vi "SetupInterfArrDev.vi"(8 "error in (no error)":errorcluster caption="entrée d'erreur (pas d'erreur)", 9 "Experiment.lvclass":refnum<class "Experiment.lvclass">=refnum, 10 "DevID":i32, 11 "Interface en entrée":refnum<class "Interface.lvclass"> caption="Interface Class in") -> (0 "error out":errorcluster caption="sortie d'erreur", 2 "CurveParamsOut":T1[](array[typedef]), 3 "Interface en sortie":refnum<class "Interface.lvclass"> caption="DNL_LabVIEW Object out")   [LabVIEW 2019, in "Interface.lvclass"]
uses:
  Interface.lvclass
  Experiment Class/Experiment.lvclass
  DevicesClass/Tools/Tools.lvclass
  CurveSetup.ctl
  SetupInterfStates.ctl
  Interface.lvclass/Interface.ctl
  2DGraphSetup.ctl
panel:
  in  "Apply All":bool
  out "InstrPref":string
  in  "SaveCurveParDef":bool
  out "GraphConfig":i32
  out "2D Scan":bool
  in  "2D Plot Act":bool caption="2D Plot"
  out "Fill Line First":bool
  in  "2D Plot":bool
  in  "2D YScanPar":u16(ring) caption="Y Parameter"
  in  "2D XScanPar":u16(ring) caption="X Parameter"
  in  "Data Only":bool
  out "GraphIndex":i32
  in  "YScale":u32(ring) items=["Left 1", "Left 2", "Left 3", "Right 1", "Right 2", "Right 3"]
  in  "X Scale":u32(ring) items=["Bottom", "Top"]
  in  "SaveCurvePar":bool
  in  "DisplayName":string
  in  "Visible":bool
  out "CrvParOut":T1[](array[typedef])
  out "NomDon":string[](array[string])=["RTêta;", "X&Y;"]
  out "VarParams":string[][](array[string])
  in  "AutoColor":bool caption="Use Automatic Color"
  out "Graphe XY":cluster{dbl, dbl}[](graph)
  in  "ScanParam":u16(ring) caption="Scan Parameter" items=["Tools.Ind Point(Point)", "Tools_1.Ind Point(Point)"]
  in  "YScaleName":string
  in  "XScaleName":string
  in  "Graph Window":i32(ring) items=["Graph 0", "No Graph", "New Graph Window For Each Curve", "New Graph Window For Each Scan"]
  in  "stop":bool
  in  "Curve List":i32(listbox)
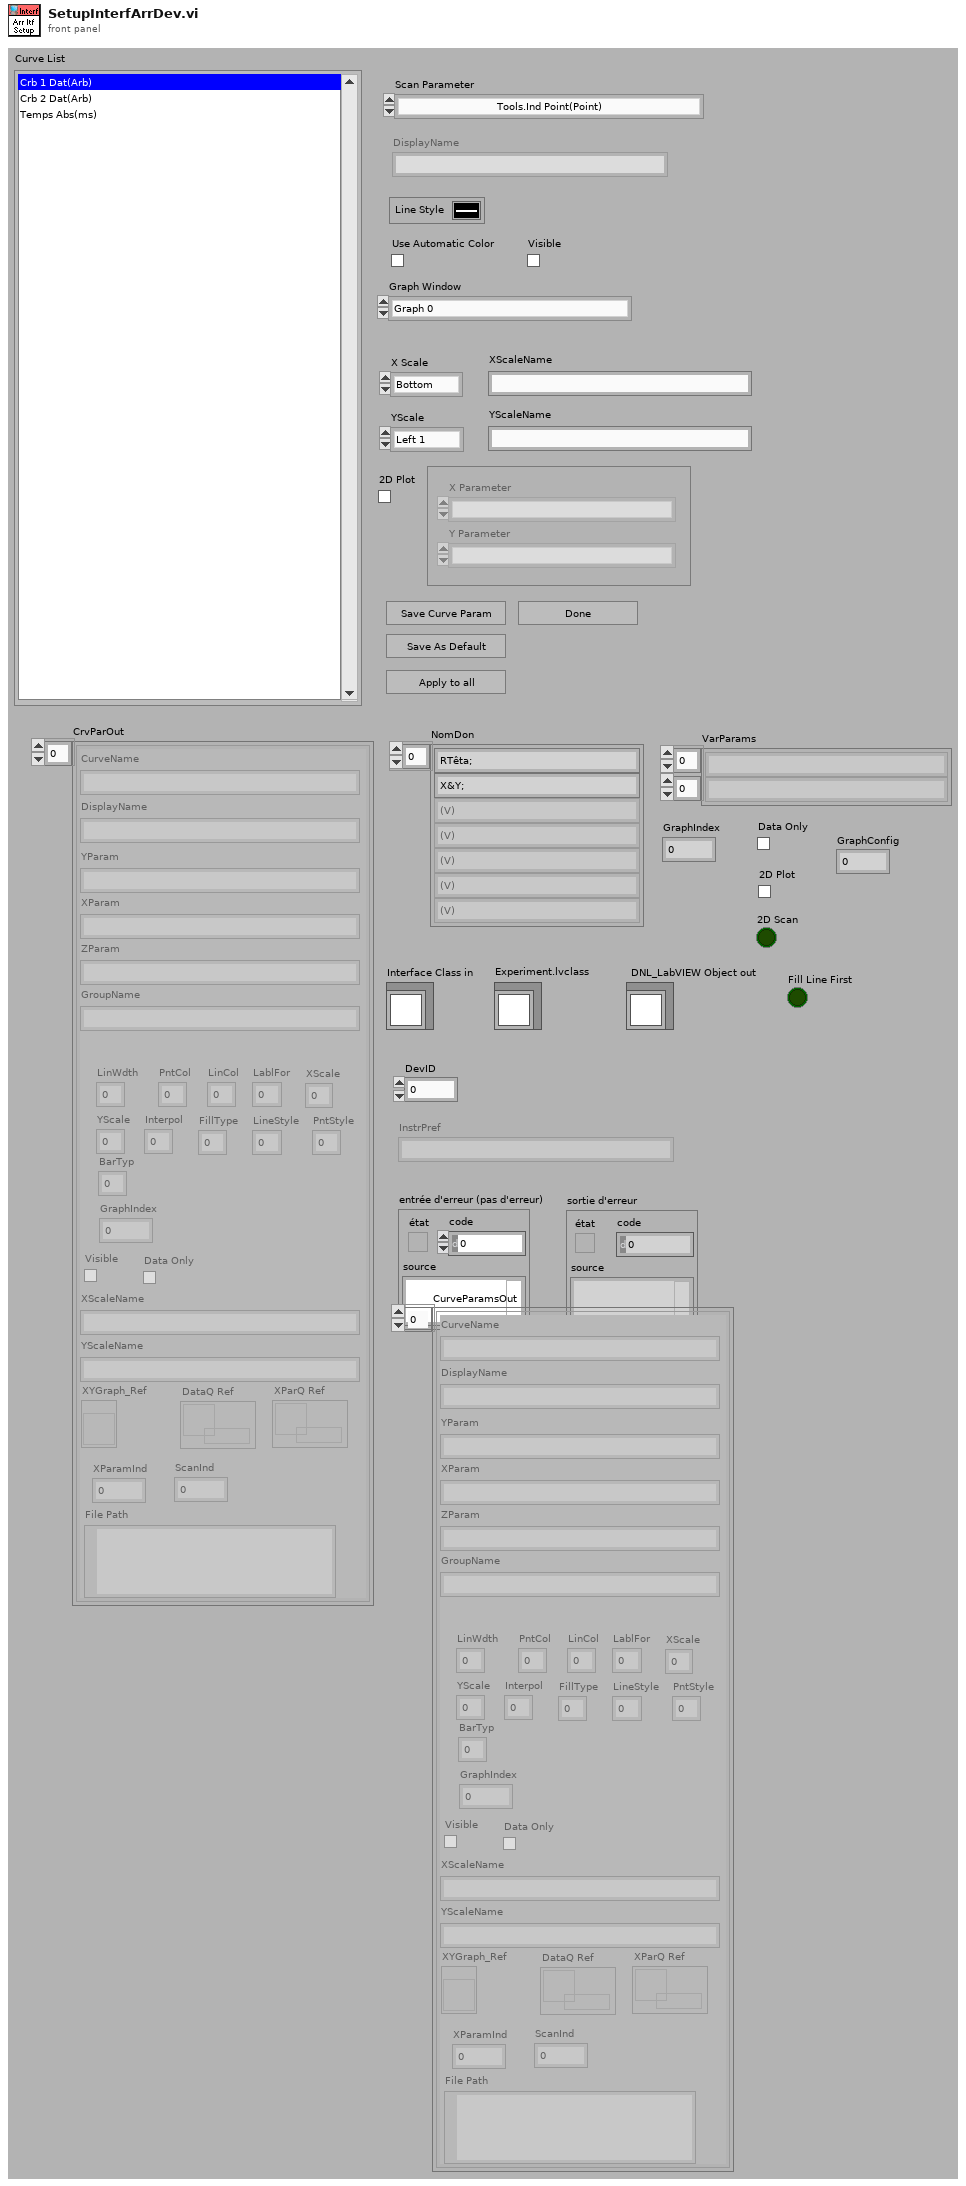
[diagram p1: front panel]
types:
  T1 = typedef "Interface.lvclass/CurveSetup.ctl" = cluster{"CurveName":string, "YParam":string, "XParam":string, "ZParam ":string, "GroupName":string, "LinWdth":u8, "PntCol":u32, "LinCol":u32, "LablFor":u8, "XScale":u32, "YScale":u32, "Interpol":u8, "DisplayName":string, "FillType":i16, "LineStyle":u8, "PntStyle":u8, "BarTyp":u8, "GraphIndex":i32, "Visible":bool, "XScaleName":string, "YScaleName":string, "XYGraph_Ref":refnum<vi>, "Data Only":bool, "DataQ Ref":refnum<queue>, "XParQ Ref":refnum<queue>, "XParamInd":i32, "ScanInd":i32, "File Path":path}
  T2 = typedef "SetupInterfStates.ctl" = enum16{"InitProg", "ReadMeasPar", "ReadCurvePar", "ReadGraphPar", "GetScaleName", "ChgScaleName", "ChngGraphConf", "2D Graph", "SaveParams", "SaveParamsDef", "ApplyAll", "ArrDevSetup", "Stop"}
  T3 = enum16{"Enable", "Disable", "DisAndGrayed", "ReinitToDefVal"}
  T4 = enum16{"Enable", "Disable", "DisAndGrayed", "ReinitToDefVal", "EnumElementsArr"}
  T5 = typedef "2DGraphSetup.ctl" = cluster{"ZDataIndex":i32, "XParIndex":i32, "YParIndex":i32, "FillLineFirst":bool, "2DGraphIndex":i32, "XParQ Ref":refnum<queue>, "YParQ Ref":refnum<queue>, "DataQRefs":refnum<queue>[], "CurveName":string, "XparInstrInd":i32, "YparInstrInd":i32, "Active":bool}
  T6 = enum32{"Invalid", "Standard", "Closed", "Hidden", "Minimized", "Maximized"}
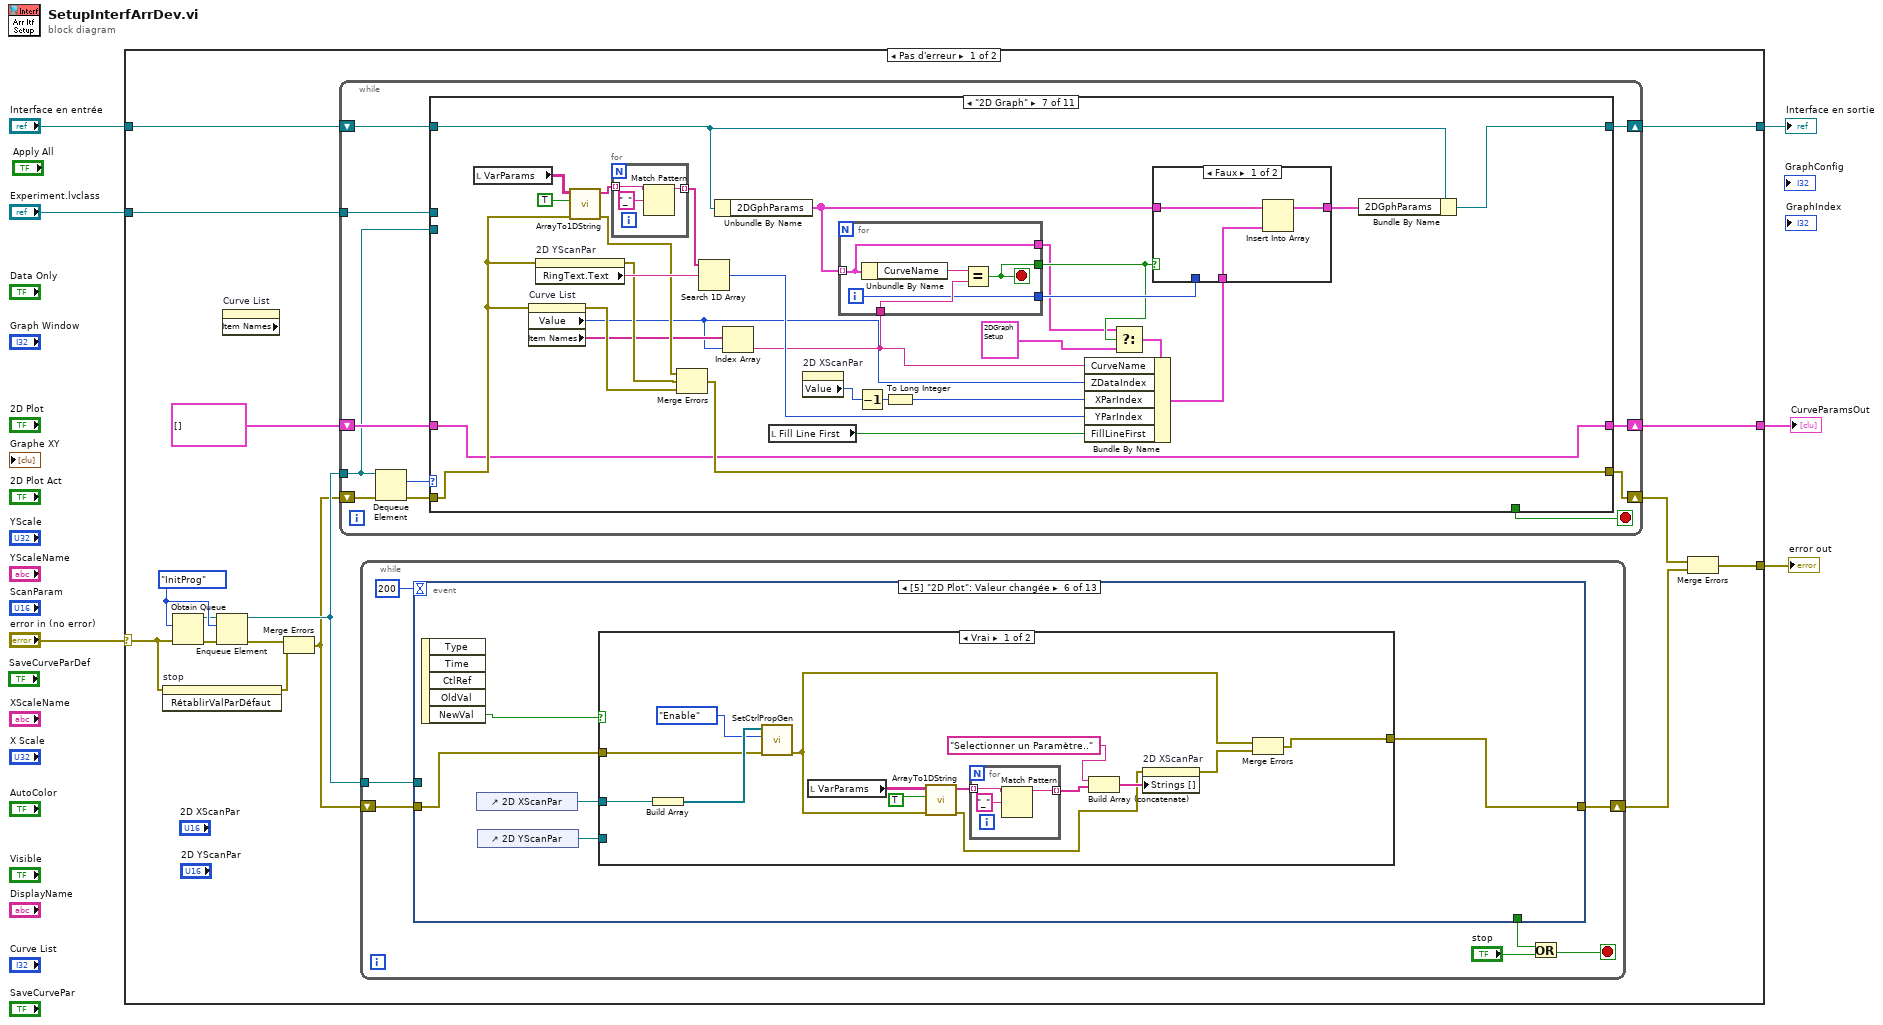
[diagram p0: block diagram]
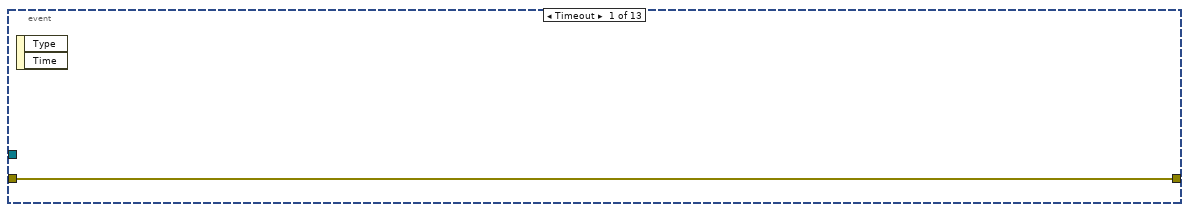
[diagram p2: hidden frame]
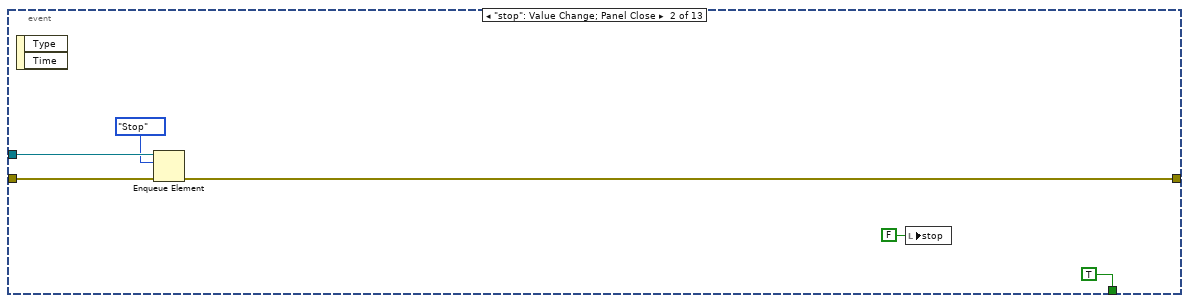
[diagram p3: hidden frame]
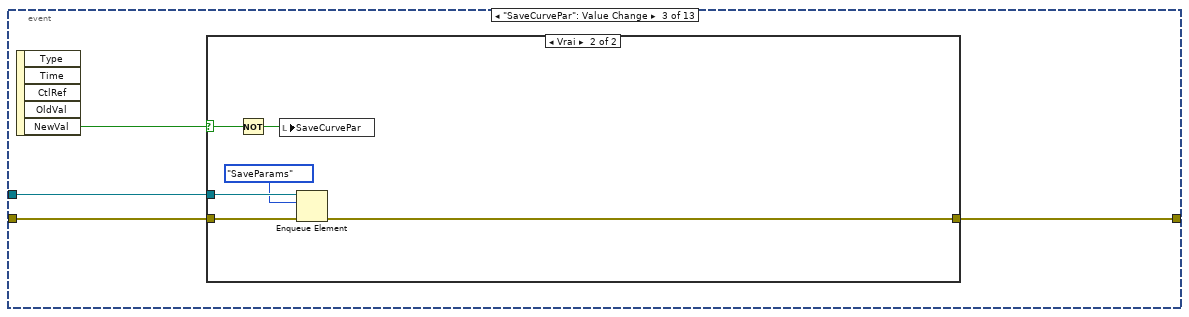
[diagram p4: hidden frame]
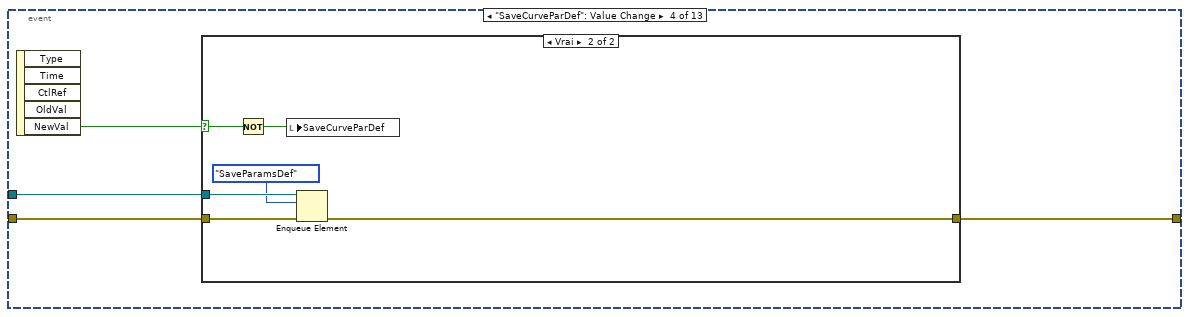
[diagram p6: hidden frame]
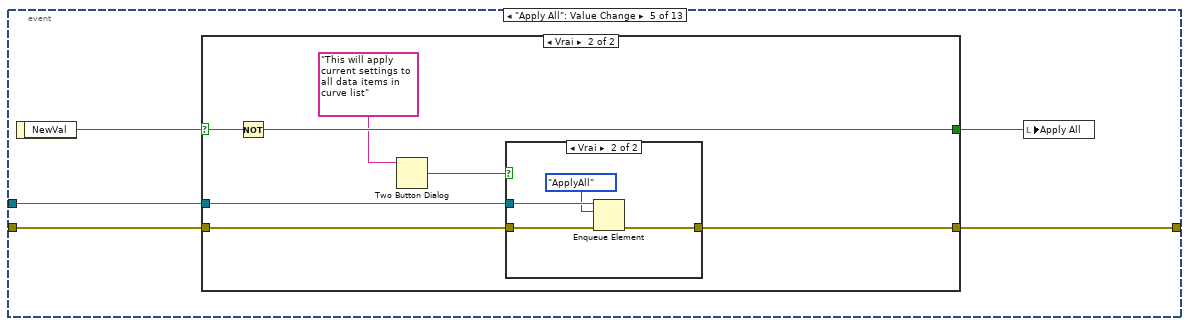
[diagram p8: hidden frame]
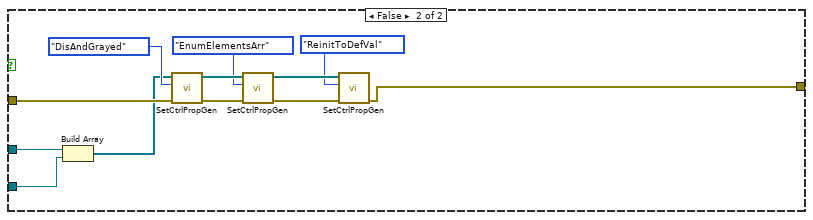
[diagram p11: hidden frame]
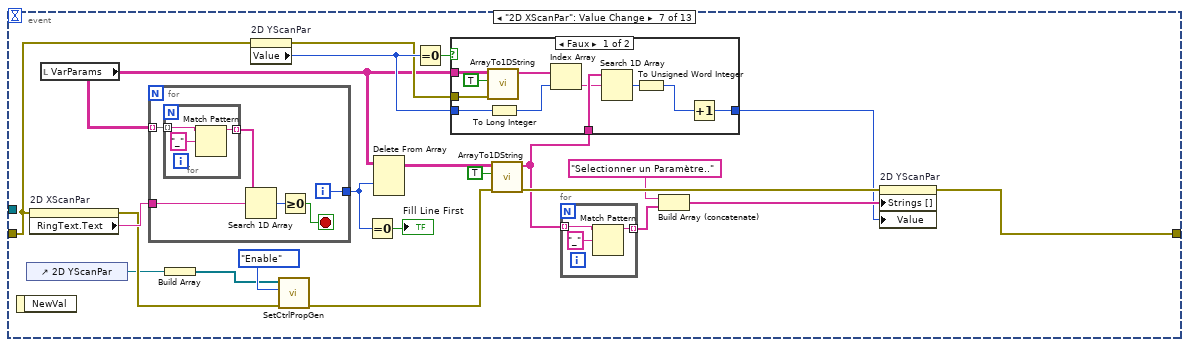
[diagram p12: hidden frame]
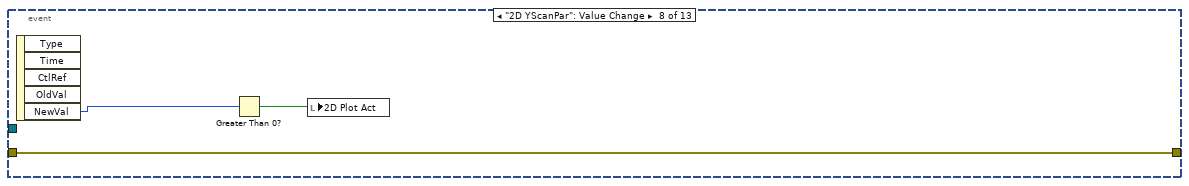
[diagram p14: hidden frame]
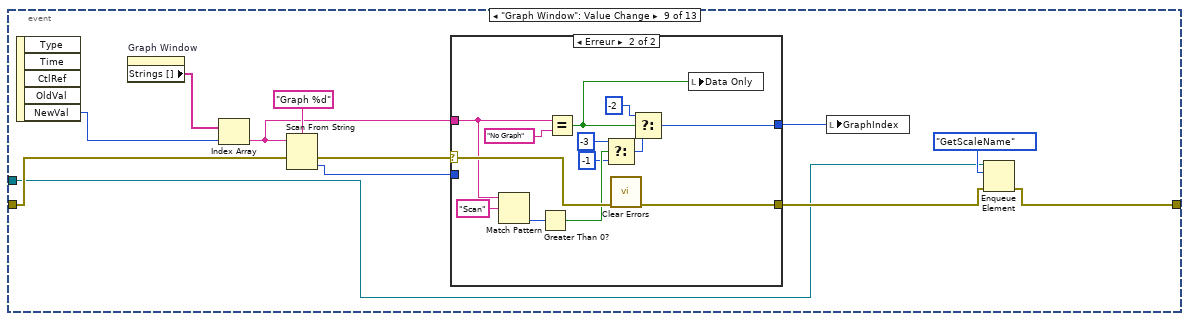
[diagram p15: hidden frame]
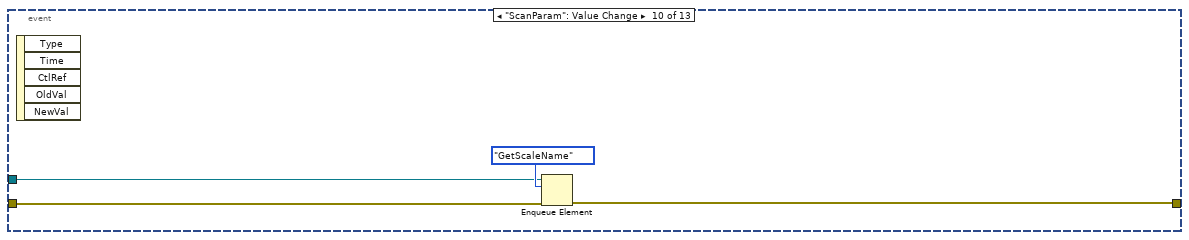
[diagram p17: hidden frame]
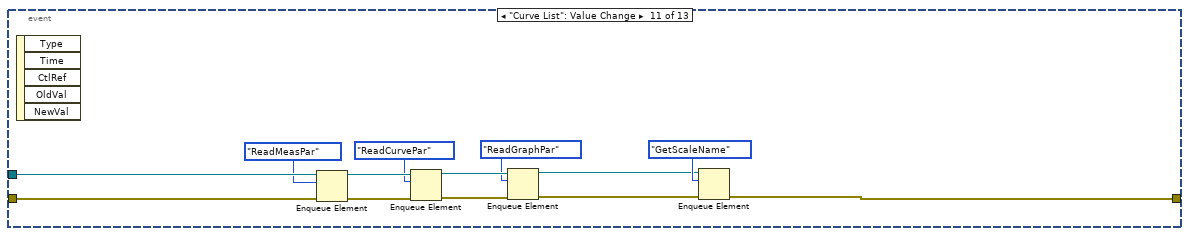
[diagram p18: hidden frame]
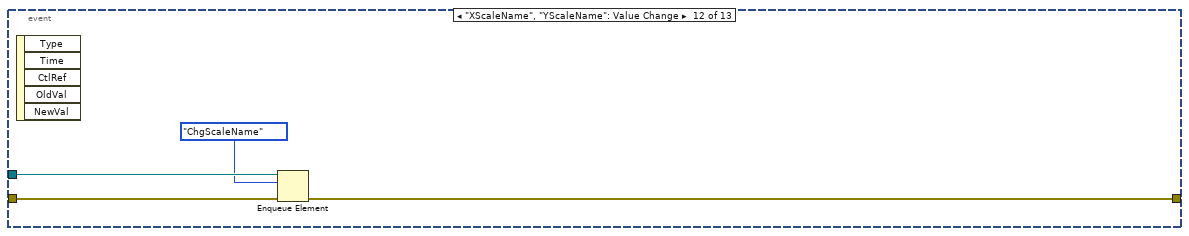
[diagram p19: hidden frame]
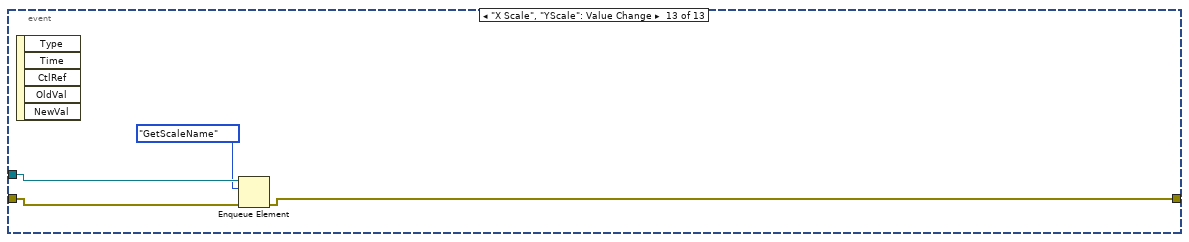
[diagram p20: hidden frame]
diagram:
  n1 = case shown="Pas d'erreur" "error in (no error)" {
    selector: "error in (no error)" -> [w17 w791]
    tunnel: [w10 w791] -> w5
    tunnel: "Interface en entrée" -> [w13 w790]
    tunnel: [w8 w790] -> w3
    tunnel: "Experiment.lvclass" -> [w9 _]
    tunnel: [w7 _] -> w1
    frame No Error {
      w22 = SetupInterfStates."InitProg" ("Énum")
      n2 = invoke on="stop" class="Bool (strict)" method="RétablirValParDéfaut"(error in=w17) -> (error out=w15:errorcluster)  [unwired: 2 in, 2 out]
      n3 = Obtain Queue(element data type=w22, error in (no error)=w17) -> (queue out=w21:refnum<queue>, error out=w20:errorcluster)  [unwired: 3 in, 1 out]
      n4 = Enqueue Element(queue=w21, element=w22, error in (no error)=w20) -> (queue out=w19:refnum<queue>, error out=w16:errorcluster)  [unwired: 1 in, 1 out]
      n5 = property on="Curve List" class="LstDér (strict)" props=["Item Names"]() -> ()  [unwired: 2 in, 3 out]
      n6 = Merge Errors(w16, w15) -> (w14:errorcluster)
      n7 = while {
        shift-right: [w217] -> w11
        shift-left: w14 -> [w222]
        tunnel: w19 -> [w214]
        shift-right: [w218] -> w8
        shift-left: w13 -> [w221]
        shift-right: [w216] -> w7
        shift-left: T1[] [] ("CurveParamsOut") -> [w215]
        tunnel: w9 -> [w213]
        stop <- w219 stop-if-true
        n8 = Dequeue Element(queue=w214, error in (no error)=w222) -> (element=w223:T2, error out=w220:errorcluster)  [unwired: 1 in, 2 out]
        n9 = case shown="\"2D Graph\"" w223 {
          tunnel: w221 -> [w227 w307 w308 w371 w443 w474 w501 w587 w614 w718 w784]
          tunnel: w220 -> [w264 w301 w331 w387 w454 w481 w503 w589 w615 w691 w778]
          tunnel: [FALSE _ _ _ _ _ _ _ _ _ TRUE] -> w219
          tunnel: [w226 w307 w308 w371 w443 w470 w500 w588 w606 w729 w784] -> w218
          tunnel: [w259 w297 w316 w358 w455 w468 w495 w590 w608 w695 w782] -> w217
          tunnel: [w225 w296 w329 w384 w465 w484 w492 w529 w605 w694 w783] -> w216
          tunnel: w215 -> [_ w296 w329 w384 w465 w484 w492 w591 w616 w692 w783]
          tunnel: w214 -> [_ _ _ _ _ _ _ w586 w613 w712 _]
          tunnel: w213 -> [w254 _ _ _ _ _ _ _ _ _ _]
          frame "InitProg", Default {
            w267 = 1 ("indice")
            # "reads the available CurveSetup or get default values"
            n10 = invoke on="2D Plot" class="Bool (strict)" method="RétablirValParDéfaut"(error in=w264) -> (error out=w251:errorcluster)  [unwired: 2 in, 2 out]
            n11 = Unbundle By Name(w227) -> ("GraphConfig"=w255:i32, "CurvesSetup"=w233:T1[], "IndCourbe"=w253:i64)
            n12 = local write "GraphConfig"(w255) -> ()
            n13 = call "ArrayDevScan.vi"("error in"=w251, "IndCourbe"=w253, "DevID"="DevID", "Experiment.lvclass In"=w254) -> ("error out"=w248:errorcluster, "ArrNomDon"=→"NomDon":string[], "ArrVarParsOut"=w249:string[][], "ArrScan list"=w245:string[], "ArrVarPar list"=w246:string[])  [unwired: 2 in, 1 out]
            "VarParams" <- w249
            n14 = Index Array(array=w245) -> (element=w244:string)  [unwired: 1 in]
            n15 = call "FormatCrvNames.vi"("entrée d'erreur"=w248, "CurveNamesIn"=w245) -> ("sortie d'erreur"=w247:errorcluster, "CurveNames"=w236:string[])  [unwired: 8 in]
            n16 = Match Pattern(string=w244, regular expression="\\.") -> (before substring=w242:string, match substring=w241:string)  [unwired: 1 in, 2 out]
            n17 = Concatenate Strings(w242, w241, "Default" ("string")) -> (w235:string)
            "InstrPref" <- w235
            n18 = for {
              tunnel: w233 -> [w289] mode=indexing
              tunnel: [w288] -> w238 mode=indexing
              n19 = Unbundle By Name(w289) -> ("CurveName"=w288:string)
            }
            n20 = call "SetCurveParams.vi"("VarPar list"=w246, "AllowDef"=TRUE, "error in (no error)"=w247, "VarParams"=w249, "CurveSetupsIn"=w233, "CurveNames"=w236) -> ("error out"=w230:errorcluster, "CurveSetupsOut"=w234:T1[])  [unwired: 4 in]
            n21 = Search 1D Array(1D array=w238, element=w235) -> (index of element=w232:i32)  [unwired: 1 in]
            n22 = Greater Or Equal To 0?(x=w232) -> (x >= 0?=w229:bool)
            n23 = case shown="Faux" w229 {
              tunnel: w236 -> [w279 w287]
              tunnel: w235 -> [_ w286]
              tunnel: w234 -> [w278 w285]
              tunnel: w233 -> [_ w284]
              tunnel: w232 -> [_ w283]
              tunnel: [w278 w281] -> w225
              tunnel: [w279 w280] -> w231
              frame False {
              }
              frame True {
                n24 = Index Array(array=w284, index=w283) -> (element=w282:T1)
                n25 = Build Array (concatenate)(w287, w286) -> (w280:string[])
                n26 = Build Array (concatenate)(w285, w282) -> (w281:T1[])
              }
            }
            "CrvParOut" <- w225
            n27 = Index Array(array=w249, index (row)=0 ("indice (ligne)")) -> (element=w272:string[])  [unwired: 1 in]
            n28 = Array Size(array=w249) -> (size(s)=w270:i32[])
            n29 = Index Array(array=w270, index=w267) -> (element=w268:i32)
            n30 = property on="Curve List" class="LstDér (strict)"(error in=w230, "Item Names"=w231) -> (error out=w271:errorcluster)  [unwired: 1 in, 1 out]
            n31 = control-ref of="2D Plot"() -> (w261:refnum<vi>)
            n32 = Greater Or Equal?(x=w268, y=w267) -> (x >= y?=w269:bool)
            "2D Scan" <- w269
            n33 = call "FormatCrvNames.vi"("entrée d'erreur"=w271, "CurveNamesIn"=w272) -> ("sortie d'erreur"=w260:errorcluster, "CurveNames"=w237:string[])  [unwired: 8 in]
            n34 = Select(t=T3."Enable" ("Énum"), s=w269, f=T3."DisAndGrayed" ("Énum")) -> (s? t:f=w265:T3)
            n35 = property on="ScanParam" class="MDér (strict)"(error in=w260, "Strings []"=w237) -> (error out=w274:errorcluster)  [unwired: 1 in, 1 out]
            n36 = Build Array(w261) -> (w263:refnum<vi>[])
            n37 = call <userlib>:"SetCtrlPropGen.vi"("Error in"=w260, "Énum"=w265, "Controls"=w263) -> ("Error out"=w256:errorcluster, "Controls Out"=w258:refnum<vi>[])  [unwired: 3 in]
            n38 = property on="Curve List" class="LstDér (strict)"(error in=w274, "Val(Sgnl)"=0 ("Valeur (Signalisation)")) -> (error out=w273:errorcluster)  [unwired: 1 in, 1 out]
            n39 = call <userlib>:"SetCtrlPropGen.vi"("Error in"=w256, "Énum"=T3."ReinitToDefVal", "Controls"=w258) -> ("Error out"=w228:errorcluster)  [unwired: 3 in, 1 out]
            n40 = call "UpdateCurveSetup.vi"("ErrorIn(No Error)"=w228, "CurveSetupsIn"=w225, "Interface.lvclass"=w227) -> ("sortie d'erreur"=w224:errorcluster, "Interface.lvclass Out"=w226:refnum<class "Interface.lvclass">)  [unwired: 7 in]
            n41 = Merge Errors(w224, w273) -> (w259:errorcluster)
          }
          frame "ReadMeasPar" {
            n42 = property on="Curve List" class="LstDér (strict)"(error in=w301) -> (error out=w298:errorcluster, "Value"=w300:i32)  [unwired: 1 in, 1 out]
            n43 = Index Array(array=w296, index=w300) -> (element=w299:T1)
            n44 = property on="ScanParam" class="MDér (strict)"(error in=w298) -> (error out=w291:errorcluster, "Strings []"=w302:string[])  [unwired: 1 in, 1 out]
            n45 = Unbundle By Name(w299) -> ("XParam"=w295:string)  [unwired: 1 out]
            n46 = Build Array(w295) -> (w294:string[])
            n47 = call "FormatCrvNames.vi"("entrée d'erreur"=w291, "CurveNamesIn"=w294) -> ("sortie d'erreur"=w290:errorcluster, "CurveNames"=w293:string[])  [unwired: 8 in]
            n48 = Index Array(array=w293) -> (element=w292:string)  [unwired: 1 in]
            n49 = Search 1D Array(1D array=w302, element=w292) -> (index of element=w305:i32)  [unwired: 1 in]
            n50 = Greater Or Equal To 0?(x=w305) -> (x >= 0?=w303:bool)
            n51 = Select(t=w305, s=w303, f=0 ("cas faux")) -> (s? t:f=w306:i32)
            n52 = property on="ScanParam" class="MDér (strict)"(error in=w290, "Value"=w306) -> (error out=w297:errorcluster)  [unwired: 1 in, 1 out]
          }
          frame "ReadCurvePar" {
            n53 = Unbundle By Name(w308) -> ("2DGphParams"=w311:T5[])
            n54 = property on="Curve List" class="LstDér (strict)"(error in=w331) -> (error out=w319:errorcluster, "Item Names"=w313:string[], "Value"=w312:i32)  [unwired: 1 in, 1 out]
            n55 = Index Array(array=w313, index=w312) -> (element=w310:string)
            n56 = Index Array(array=w329, index=w312) -> (element=w332:T1)
            n57 = for {
              tunnel: w311 -> [w341] mode=indexing
              tunnel: w310 -> [w343]
              tunnel: [w342] -> _
              tunnel: [w341] -> w309
              stop <- w342 stop-if-true
              n58 = Unbundle By Name(w341) -> ("CurveName"=w344:string)
              n59 = Equal?(x=w344, y=w343) -> (x = y?=w342:bool)
            }
            n60 = Unbundle By Name(w332) -> ("PntCol"=w328:u32, "LinCol"=w327:u32)
            n61 = Unbundle By Name(w332) -> ("LinWdth"=w340:u8, "LablFor"=w334:u8)
            n62 = Unbundle By Name(w332) -> ("Interpol"=w335:u8, "FillType"=w336:i16, "LineStyle"=w337:u8, "PntStyle"=w338:u8, "BarTyp"=w339:u8)
            n63 = call "GetPlotColors.vi"("Color2In"=w327, "Color1In"=w328, "ColorIndex"=0) -> ("Color2Out"=w323:u32, "Color1Out"=w324:u32, "AutoColor"=w325:bool)  [unwired: 5 in, 1 out]
            n64 = local write "AutoColor"(w325) -> ()
            n65 = property on="Graphe XY" class="GraphXY (strict)"(error in=w319, "Active Plot"=u32 0 ("Tracé actif"), "Plot.Fill/Pt. Color"=w324, "Plot.Plot Color"=w323, "Plot.Line Width"=w340, "Plot.Label Style"=w334, "Plot.Plot Interpolation"=w335, "Plot.Fill To"=w336, "Plot.Line Style"=w337, "Plot.Point Style"=w338, "Plot.Bar Plot Style"=w339) -> (error out=w330:errorcluster)  [unwired: 1 in, 1 out]
            n66 = Unbundle By Name(w309) -> ("ZDataIndex"=w320:i32, "XParIndex"=w318:i32, "YParIndex"=w317:i32)
            n67 = Greater Or Equal To 0?(x=w320) -> (x >= 0?=w314:bool)
            n68 = call <vilib>:"General Error Handler.vi"("error in (no error)"=w330) -> ("error out"=w322:errorcluster)  [unwired: 10 in, 4 out]
            n69 = case shown="Vrai" w314 {
              tunnel: w320 -> [_ _]
              tunnel: w319 -> [w346 w353]
              tunnel: w318 -> [_ w356]
              tunnel: w317 -> [_ w348]
              tunnel: [w345 w350] -> w315
              frame False {
                n70 = property on="2D Plot" class="Bool (strict)"(error in=w346, "Val(Sgnl)"=FALSE ("Valeur (Signalisation)")) -> (error out=w345:errorcluster)  [unwired: 1 in, 1 out]
              }
              frame True {
                n71 = property on="2D Plot" class="Bool (strict)"(error in=w353, "Val(Sgnl)"=TRUE ("Valeur (Signalisation)")) -> (error out=w357:errorcluster)  [unwired: 1 in, 1 out]
                n72 = Increment(x=w356) -> (x+1=w355:i32)
                n73 = To Unsigned Word Integer(number=w355) -> (unsigned 16bit integer=w354:u16)
                n74 = property on="2D XScanPar" class="MDér (strict)"(error in=w357, "Val(Sgnl)"=w354) -> (error out=w352:errorcluster)  [unwired: 1 in, 1 out]
                n75 = To Unsigned Word Integer(number=w348) -> (unsigned 16bit integer=w351:u16)
                n76 = property on="2D YScanPar" class="MDér (strict)"(error in=w352, "Value"=w351) -> (error out=w350:errorcluster)  [unwired: 1 in, 1 out]
              }
            }
            n77 = local write "2D Plot Act"(w314) -> ()
            n78 = call <vilib>:"Clear Errors.vi"("error in (no error)"=w322) -> ("error out"=w321:errorcluster)  [unwired: 5 in, 1 out]
            n79 = Merge Errors(w315, w321) -> (w316:errorcluster)
          }
          frame "ReadGraphPar" {
            n80 = local read "GraphConfig"() -> (w364:i32)
            n81 = property on="Curve List" class="LstDér (strict)"(error in=w387) -> (error out=w378:errorcluster, "Value"=w370:i32)  [unwired: 1 in, 1 out]
            n82 = Index Array(array=w384, index=w370) -> (element=w385:T1)
            n83 = local read "2D Scan"() -> (w360:bool)
            n84 = Unbundle By Name(w385) -> ("GraphIndex"=w379:i32)
            n85 = call "GraphConfCount.vi"("Configuration"=w364) -> ("GraphCount"=w363:i32)  [unwired: 9 in, 1 out]
            n86 = To Long Integer(number=w363) -> (32bit integer=w380:i32)
            n87 = Greater Or Equal To 0?(x=w379) -> (x >= 0?=w381:bool)
            n88 = Select(t=string[] ["No Graph", "New Graph Window For Each Curve", "New Graph Window For Each Scan"], s=w360, f=string[] ["No Graph", "New Graph Window "]) -> (s? t:f=w362:string[])
            n89 = case shown="Vrai" w381 {
              tunnel: w380 -> [w390 w417]
              tunnel: w379 -> [w388 w419]
              tunnel: [w395 w422] -> w377
              tunnel: w378 -> [w394 w421]
              tunnel: [w392 w420] -> w376
              tunnel: w362 -> [w391 w416]
              tunnel: [w393 w418] -> w375
              tunnel: [w389 w415] -> w374
              frame False {
                # "either new window (-1,-3) or no window(-2)"
                n90 = Equal?(x=w388, y=-2) -> (x = y?=w396:bool)
                n91 = case shown="Faux" w396 {
                  tunnel: [w408 w414] -> w395
                  tunnel: w394 -> [w408 w414]
                  tunnel: w390 -> [w407 w413]
                  tunnel: [w410 w413] -> w393
                  tunnel: [w409 w412] -> w392
                  tunnel: w391 -> [w409 w412]
                  tunnel: [w400 -2] -> w389
                  tunnel: w388 -> [w406 _]
                  frame False {
                    n92 = Equal?(x=w406, y=-1) -> (x = y?=w401:bool)
                    n93 = Select(t=1 ("y"), s=w401, f=2 ("y")) -> (s? t:f=w402:i32)
                    n94 = Select(t=-1, s=w401, f=-3) -> (s? t:f=w400:i32)
                    n95 = Add(x=w407, y=w402) -> (x+y=w410:i32)
                  }
                  frame True {
                    # "No graph"
                  }
                }
              }
              frame True {
                # "either valid or invalid (absent) graph window"
                n96 = Less Or Equal?(x=w417, y=w419) -> (x <= y?=w423:bool)
                n97 = case shown="Vrai" w423 {
                  tunnel: w421 -> [w426 w435]
                  tunnel: [w426 w434] -> w422
                  tunnel: [w425 w432] -> w420
                  tunnel: w416 -> [w425 w431]
                  tunnel: w419 -> [w424 w427]
                  tunnel: [w424 w428] -> w418
                  tunnel: w417 -> [_ w430]
                  tunnel: [w424 w427] -> w415
                  frame False {
                  }
                  frame True {
                    n98 = Add(x=w430, y=2) -> (x+y=w428:i32)
                    n99 = Format Into String(format string="Graph %d (unavailable)" ("chaîne de format"), error in=w435, w427) -> (resulting string=w433:string, error out=w434:errorcluster)  [unwired: 1 in]
                    n100 = Build Array (concatenate)(w431, w433) -> (w432:string[])
                  }
                }
              }
            }
            n101 = for {
              N: w380 -> [_]
              tunnel: [w437] -> w383 mode=indexing
              i -> [w439]
              n102 = Format Into String(format string="Graph %d" ("chaîne de format"), w439) -> (resulting string=w437:string)  [unwired: 2 in, 1 out]
            }
            n103 = local write "GraphIndex"(w374) -> ()
            n104 = Unbundle By Name(w385) -> ("Data Only"=w372:bool, "DisplayName"=w373:string, "Visible"=w386:bool, "XScale"=w367:u32, "YScale"=w366:u32)
            n105 = Build Array (concatenate)(w383, w376) -> (w382:string[])
            n106 = property on="Graph Window" class="MDér (strict)"(error in=w377, "Strings []"=w382, "Value"=w375) -> (error out=w365:errorcluster)  [unwired: 1 in, 1 out]
            n107 = local write "Data Only"(w372) -> ()
            n108 = local write "DisplayName"(w373) -> ()
            n109 = local write "Visible"(w386) -> ()
            n110 = property on="X Scale" class="MDér (strict)"(error in=w365, "Value"=w367) -> (error out=w369:errorcluster)  [unwired: 1 in, 1 out]
            n111 = property on="YScale" class="MDér (strict)"(error in=w365, "Value"=w366) -> (error out=w368:errorcluster)  [unwired: 1 in, 1 out]
            n112 = Merge Errors(w369, w368) -> (w358:errorcluster)
          }
          frame "GetScaleName" {
            # "if you don't \"save param\"\ngraph stays with no scale"
            # "The first data element gives is names to the y scale #0\nThe first varpar gives is name to the x scale #0\nOther scale number get their names attributed at selection"
            n113 = property on="GraphIndex" class="NumNb (strict)"(error in=w454) -> ("Value"=w449:i32)  [unwired: 1 in, 2 out]
            n114 = property on="Curve List" class="LstDér (strict)"(error in=w454) -> (error out=w441:errorcluster, "Value"=w466:i32)  [unwired: 1 in, 1 out]
            n115 = Index Array(array=w465, index=w466) -> (element=w461:T1)
            n116 = property on="ScanParam" class="MDér (strict)"(error in=w441) -> (error out=w440:errorcluster, "RingText.Text"=w442:string)  [unwired: 1 in, 1 out]
            n117 = Unbundle By Name(w461) -> ("CurveName"=w458:string)
            n118 = property on="X Scale" class="MDér (strict)"(error in=w441) -> (error out=w457:errorcluster, "Value"=w452:u32)  [unwired: 1 in, 1 out]
            n119 = property on="YScale" class="MDér (strict)"(error in=w441) -> (error out=w456:errorcluster, "Value"=w447:u32)  [unwired: 1 in, 1 out]
            n120 = Unbundle By Name(w443) -> ("XScalesNames"=w453:string[][], "YScalesNames"=w448:string[][])
            n121 = Merge Errors(w440, w457, w456) -> (w455:errorcluster)
            n122 = Index Array(array=w448, index (row)=w449, index (col)=w447) -> (element=w446:string)
            n123 = Index Array(array=w453, index (row)=w449, index (col)=w452) -> (element=w463:string)
            n124 = Match Pattern(string=w458, regular expression="_" ("expression régulière")) -> (before substring=w459:string)  [unwired: 1 in, 3 out]
            n125 = Match Pattern(string=w442, regular expression="_" ("expression régulière")) -> (before substring=w460:string)  [unwired: 1 in, 3 out]
            n126 = Empty String/Path?(string/path=w463) -> (empty?=w445:bool)
            n127 = Empty String/Path?(string/path=w446) -> (empty?=w444:bool)
            n128 = Select(t=w459, s=w444, f=w446) -> (s? t:f=w450:string)
            n129 = Select(t=w460, s=w445, f=w463) -> (s? t:f=w451:string)
            n130 = local write "YScaleName"(w450) -> ()
            n131 = local write "XScaleName"(w451) -> ()
          }
          frame "ChgScaleName" {
            n132 = Unbundle By Name(w474) -> ("XScalesNames"=w478:string[][], "YScalesNames"=w477:string[][])
            n133 = property on="X Scale" class="MDér (strict)"(error in=w481) -> (error out=w473:errorcluster, "Value"=w480:u32)  [unwired: 1 in, 1 out]
            n134 = property on="YScale" class="MDér (strict)"(error in=w481) -> (error out=w472:errorcluster, "Value"=w479:u32)  [unwired: 1 in, 1 out]
            n135 = Merge Errors(w473, w472) -> (w467:errorcluster)
            n136 = local read "GraphIndex"() -> (w469:i32)
            n137 = local read "YScaleName"() -> (w483:string)
            n138 = local read "XScaleName"() -> (w482:string)
            n139 = Replace Array Subset(array=w478, new element=w482, index (row)=w469, index (col)=w480) -> (w475:string[][])
            n140 = Replace Array Subset(array=w477, new element=w483, index (row)=w469, index (col)=w479) -> (w476:string[][])
            n141 = Bundle By Name(cluster=w474, "XScalesNames"=w475, "YScalesNames"=w476) -> (w471:refnum<class "Interface.lvclass">)
            n142 = call "SetGrphScale.vi"("error in (no error)"=w467, "GraphIndex"=w469, "Interface en entrée"=w471) -> ("error out"=w468:errorcluster, "Interface en sortie"=w470:refnum<class "Interface.lvclass">)  [unwired: 7 in]
          }
          frame "2D Graph" {
            n143 = local read "VarParams"() -> (w509:string[][])
            n144 = property on="Curve List" class="LstDér (strict)"(error in=w503) -> (error out=w496:errorcluster, "Value"=w493:i32, "Item Names"=w494:string[])  [unwired: 1 in, 1 out]
            n145 = property on="2D YScanPar" class="MDér (strict)"(error in=w503) -> (error out=w497:errorcluster, "RingText.Text"=w507:string)  [unwired: 1 in, 1 out]
            n146 = call <userlib>:"ArrayTo1DString.vi"("ErrorIn(No Error)"=w503, "DelArrEnd(F)"=TRUE ("DelArrEnd"), "tableau"=w509) -> ("sortie d'erreur"=w498:errorcluster, "Array Out"=w508:string[])  [unwired: 6 in, 1 out]
            n147 = for {
              tunnel: w508 -> [w528] mode=indexing
              tunnel: [w527] -> w506 mode=indexing
              n148 = Match Pattern(string=w528, regular expression="_" ("expression régulière")) -> (before substring=w527:string)  [unwired: 1 in, 3 out]
            }
            n149 = Merge Errors(w498, w497, w496) -> (w495:errorcluster)
            n150 = Search 1D Array(1D array=w506, element=w507) -> (index of element=w505:i32)  [unwired: 1 in]
            n151 = Unbundle By Name(w501) -> ("2DGphParams"=w490:T5[])
            n152 = Index Array(array=w494, index=w493) -> (element=w491:string)
            n153 = local read "Fill Line First"() -> (w511:bool)
            n154 = property on="2D XScanPar" class="MDér (strict)"() -> ("Value"=w513:u16)  [unwired: 2 in, 2 out]
            n155 = for {
              tunnel: w490 -> [w514] mode=indexing
              tunnel: w491 -> [w517]
              tunnel: [w516] -> w488
              tunnel: [w514] -> w487
              tunnel: [w515] -> w489
              i -> [w515]
              stop <- w516 stop-if-true
              n156 = Unbundle By Name(w514) -> ("CurveName"=w518:string)
              n157 = Equal?(x=w518, y=w517) -> (x = y?=w516:bool)
            }
            n158 = Decrement(x=w513) -> (x-1=w512:u16)
            n159 = To Long Integer(number=w512) -> (32bit integer=w504:i32)
            n160 = Select(t=w487, s=w488, f=T5 {"ZDataIndex"=-1, "XParIndex"=-1, "YParIndex"=-1, "FillLineFirst"=FALSE, "2DGraphIndex"=0, "XParQ Ref"=refnum, "YParQ Ref"=refnum, "DataQRefs"=[], "CurveName"="", "XparInstrInd"=-1, "YparInstrInd"=-1, "Active"=FALSE} ("cas faux")) -> (s? t:f=w486:T5)
            n161 = Bundle By Name(cluster=w486, "CurveName"=w491, "ZDataIndex"=w493, "XParIndex"=w504, "YParIndex"=w505, "FillLineFirst"=w511) -> (w502:T5)
            n162 = case shown="Faux" w488 {
              tunnel: w490 -> [w521 w525]
              tunnel: w502 -> [w520 w522]
              tunnel: [w519 w524] -> w499
              tunnel: w489 -> [_ w523]
              frame False {
                n163 = Insert Into Array(array=w521, new element=w520) -> (w519:T5[])  [unwired: 1 in]
              }
              frame True {
                n164 = Replace Array Subset(array=w525, new element=w522, index=w523) -> (w524:T5[])
              }
            }
            n165 = Bundle By Name(cluster=w501, "2DGphParams"=w499) -> (w500:refnum<class "Interface.lvclass">)
          }
          frame "SaveParams" {
            n166 = local read "2D Plot Act"() -> (w585:bool)
            n167 = property on="Curve List" class="LstDér (strict)"(error in=w589) -> (error out=w584:errorcluster, "Value"=w534:i32)  [unwired: 1 in, 1 out]
            n168 = local read "GraphIndex"() -> (w539:i32)
            n169 = Unbundle By Name(w587) -> ("XScalesNames"=w547:string[][], "YScalesNames"=w546:string[][])
            n170 = Index Array(array=w591, index=w534) -> (element=w575:T1)
            n171 = case shown="Vrai" w585 {
              tunnel: w586 -> [_ w595]
              tunnel: w584 -> [w592 w594]
              tunnel: [w592 w593] -> w536
              frame False {
              }
              frame True {
                n172 = Enqueue Element(queue=w595, element=SetupInterfStates."2D Graph" ("Énum"), error in (no error)=w594) -> (error out=w593:errorcluster)  [unwired: 1 in, 2 out]
              }
            }
            n173 = local read "YScaleName"() -> (w548:string)
            n174 = property on="X Scale" class="MDér (strict)"(error in=w584) -> (error out=w553:errorcluster, "Value"=w545:u32)  [unwired: 1 in, 1 out]
            n175 = local read "XScaleName"() -> (w549:string)
            n176 = property on="YScale" class="MDér (strict)"(error in=w553) -> (error out=w540:errorcluster, "Value"=w544:u32)  [unwired: 1 in, 1 out]
            n177 = Replace Array Subset(array=w546, new element=w548, index (row)=w539, index (col)=w544) -> (w542:string[][])
            n178 = Replace Array Subset(array=w547, new element=w549, index (row)=w539, index (col)=w545) -> (w543:string[][])
            n179 = Bundle By Name(cluster=w575, "XScale"=w545, "YScale"=w544, "GraphIndex"=w539) -> (w574:T1)
            n180 = Merge Errors(w536, w540) -> (w537:errorcluster)
            n181 = Bundle By Name(cluster=w587, "XScalesNames"=w543, "YScalesNames"=w542) -> (w541:refnum<class "Interface.lvclass">)
            n182 = property on="Graphe XY" class="GraphXY (strict)"(error in=w537, "Active Plot"=u32 0 ("Tracé actif")) -> (error out=w564:errorcluster, "Plot.Fill/Pt. Color"=w572:u32, "Plot.Plot Color"=w571:u32, "Plot.Line Width"=w582:u8, "Plot.Label Style"=w581:u8, "Plot.Plot Interpolation"=w580:u8, "Plot.Fill To"=w579:i16, "Plot.Line Style"=w578:u8, "Plot.Point Style"=w577:u8, "Plot.Bar Plot Style"=w576:u8)  [unwired: 1 in, 1 out]
            n183 = local read "AutoColor"() -> (w573:bool)
            n184 = call "SetGrphScale.vi"("error in (no error)"=w537, "GraphIndex"=w539, "Interface en entrée"=w541) -> ("error out"=w533:errorcluster, "Interface en sortie"=w531:refnum<class "Interface.lvclass">)  [unwired: 7 in]
            n185 = case shown="Vrai" w573 {
              tunnel: w574 -> [w602 w604]
              tunnel: w572 -> [w601 _]
              tunnel: w571 -> [w598 _]
              tunnel: [w600 w604] -> w559
              frame False {
                n186 = To Long Integer(number=w601) -> (32bit integer=w599:i32)
                n187 = To Long Integer(number=w598) -> (32bit integer=w597:i32)
                n188 = Bundle By Name(cluster=w602, "PntCol"=w599, "LinCol"=w597) -> (w600:T1)
              }
              frame True {
                w603 = -1 ("PntCol")
                n189 = Bundle By Name(cluster=w604, "PntCol"=w603, "LinCol"=w603) -> ()  [unwired: 1 out]
              }
            }
            n190 = Bundle By Name(cluster=w559, "LinWdth"=w582, "LablFor"=w581, "Interpol"=w580, "FillType"=w579, "LineStyle"=w578, "PntStyle"=w577, "BarTyp"=w576) -> (w566:T1)
            n191 = local read "VarParams"() -> (w557:string[][])
            n192 = property on="ScanParam" class="MDér (strict)"(error in=w564) -> (error out=w560:errorcluster, "Value"=w555:u16)  [unwired: 1 in, 1 out]
            n193 = property on="Curve List" class="LstDér (strict)"(error in=w564) -> (error out=w552:errorcluster, "Item Names"=w563:string[], "Value"=w562:i32)  [unwired: 1 in, 1 out]
            n194 = local read "DisplayName"() -> (w535:string)
            n195 = local read "Visible"() -> (w570:bool)
            n196 = local read "XScaleName"() -> (w569:string)
            n197 = local read "YScaleName"() -> (w568:string)
            n198 = local read "Data Only"() -> (w550:bool)
            n199 = Index Array(array=w557, index (row)=0 ("indice (ligne)")) -> (element=w558:string[])  [unwired: 1 in]
            n200 = To Long Integer(number=w555) -> (32bit integer=w538:i32)
            n201 = Index Array(array=w563, index=w562) -> (element=w561:string)
            n202 = Index Array(array=w558, index=w538) -> (element=w554:string)
            n203 = local read "GraphConfig"() -> (w551:i32)
            n204 = Bundle By Name(cluster=w566, "CurveName"=w561, "XParam"=w554, "XParamInd"=w538) -> (w565:T1)
            n205 = Bundle By Name(cluster=w565, "DisplayName"=w535, "Visible"=w570, "XScaleName"=w569, "YScaleName"=w568, "Data Only"=w550) -> (w567:T1)
            n206 = Replace Array Subset(array=w591, new element=w567, index=w534) -> (w529:T1[])
            n207 = call "UpdateCurveSetup.vi"("ErrorIn(No Error)"=w533, "CurveSetupsIn"=w529, "Interface.lvclass"=w531) -> ("sortie d'erreur"=w532:errorcluster, "Interface.lvclass Out"=w530:refnum<class "Interface.lvclass">)  [unwired: 7 in]
            n208 = Bundle By Name(cluster=w530, "GraphConfig"=w551) -> (w588:refnum<class "Interface.lvclass">)
            n209 = Merge Errors(w552, w560, w532) -> (w590:errorcluster)
          }
          frame "ApplyAll" {
            n210 = local read "2D Plot Act"() -> (w612:bool)
            n211 = property on="Curve List" class="LstDér (strict)"(error in=w615) -> (error out=w611:errorcluster, "Item Names"=w610:string[])  [unwired: 1 in, 1 out]
            n212 = for {
              tunnel: w613 -> [w624]
              tunnel: w612 -> [w623]
              shift-right: [w643] -> w607
              shift-left: w614 -> [w631]
              shift-right: [w652] -> w609
              shift-left: w611 -> [w622]
              shift-right: [w617] -> w605
              shift-left: w616 -> [w660]
              tunnel: w610 -> [_] mode=indexing
              i -> [w618]
              n213 = local read "GraphIndex"() -> (w626:i32)
              n214 = Unbundle By Name(w631) -> ("XScalesNames"=w637:string[][], "YScalesNames"=w636:string[][])
              n215 = Index Array(array=w660, index=w618) -> (element=w668:T1)
              n216 = case shown="Vrai" w623 {
                tunnel: w624 -> [_ w680]
                tunnel: w622 -> [w677 w679]
                tunnel: [w677 w678] -> w620
                frame False {
                }
                frame True {
                  n217 = Enqueue Element(queue=w680, element=SetupInterfStates."2D Graph" ("Énum"), error in (no error)=w679) -> (error out=w678:errorcluster)  [unwired: 1 in, 2 out]
                }
              }
              n218 = local read "YScaleName"() -> (w638:string)
              n219 = property on="X Scale" class="MDér (strict)"(error in=w622) -> (error out=w644:errorcluster, "Value"=w635:u32)  [unwired: 1 in, 1 out]
              n220 = local read "XScaleName"() -> (w639:string)
              n221 = property on="YScale" class="MDér (strict)"(error in=w644) -> (error out=w629:errorcluster, "Value"=w634:u32)  [unwired: 1 in, 1 out]
              n222 = Replace Array Subset(array=w636, new element=w638, index (row)=w626, index (col)=w634) -> (w632:string[][])
              n223 = Replace Array Subset(array=w637, new element=w639, index (row)=w626, index (col)=w635) -> (w633:string[][])
              n224 = Bundle By Name(cluster=w668, "XScale"=w635, "YScale"=w634, "GraphIndex"=w626) -> (w667:T1)
              n225 = Merge Errors(w620, w629) -> (w621:errorcluster)
              n226 = Bundle By Name(cluster=w631, "XScalesNames"=w633, "YScalesNames"=w632) -> (w630:refnum<class "Interface.lvclass">)
              n227 = property on="Graphe XY" class="GraphXY (strict)"(error in=w621, "Active Plot"=u32 0 ("Tracé actif")) -> (error out=w656:errorcluster, "Plot.Fill/Pt. Color"=w665:u32, "Plot.Plot Color"=w664:u32, "Plot.Line Width"=w675:u8, "Plot.Label Style"=w674:u8, "Plot.Plot Interpolation"=w673:u8, "Plot.Fill To"=w672:i16, "Plot.Line Style"=w671:u8, "Plot.Point Style"=w670:u8, "Plot.Bar Plot Style"=w669:u8)  [unwired: 1 in, 1 out]
              n228 = local read "AutoColor"() -> (w666:bool)
              n229 = call "SetGrphScale.vi"("error in (no error)"=w621, "GraphIndex"=w626, "Interface en entrée"=w630) -> ("error out"=w627:errorcluster, "Interface en sortie"=w628:refnum<class "Interface.lvclass">)  [unwired: 7 in]
              n230 = case shown="Vrai" w666 {
                tunnel: w667 -> [w687 w689]
                tunnel: w665 -> [w686 _]
                tunnel: w664 -> [w683 _]
                tunnel: [w685 w689] -> w650
                frame False {
                  n231 = To Long Integer(number=w686) -> (32bit integer=w684:i32)
                  n232 = To Long Integer(number=w683) -> (32bit integer=w682:i32)
                  n233 = Bundle By Name(cluster=w687, "PntCol"=w684, "LinCol"=w682) -> (w685:T1)
                }
                frame True {
                  w688 = -1 ("PntCol")
                  n234 = Bundle By Name(cluster=w689, "PntCol"=w688, "LinCol"=w688) -> ()  [unwired: 1 out]
                }
              }
              n235 = Bundle By Name(cluster=w650, "LinWdth"=w675, "LablFor"=w674, "Interpol"=w673, "FillType"=w672, "LineStyle"=w671, "PntStyle"=w670, "BarTyp"=w669) -> (w658:T1)
              n236 = local read "VarParams"() -> (w648:string[][])
              n237 = property on="ScanParam" class="MDér (strict)"(error in=w656) -> (error out=w651:errorcluster, "Value"=w646:u16)  [unwired: 1 in, 1 out]
              n238 = property on="Curve List" class="LstDér (strict)"(error in=w656) -> (error out=w642:errorcluster, "Item Names"=w655:string[], "Value"=w654:i32)  [unwired: 1 in, 1 out]
              n239 = local read "DisplayName"() -> (w619:string)
              n240 = local read "Visible"() -> (w663:bool)
              n241 = local read "XScaleName"() -> (w662:string)
              n242 = local read "YScaleName"() -> (w661:string)
              n243 = local read "Data Only"() -> (w640:bool)
              n244 = Index Array(array=w648, index (row)=0 ("indice (ligne)")) -> (element=w649:string[])  [unwired: 1 in]
              n245 = To Long Integer(number=w646) -> (32bit integer=w625:i32)
              n246 = Index Array(array=w655, index=w654) -> (element=w653:string)
              n247 = Index Array(array=w649, index=w625) -> (element=w645:string)
              n248 = local read "GraphConfig"() -> (w641:i32)
              n249 = Bundle By Name(cluster=w658, "CurveName"=w653, "XParam"=w645, "XParamInd"=w625) -> (w657:T1)
              n250 = Bundle By Name(cluster=w657, "DisplayName"=w619, "Visible"=w663, "XScaleName"=w662, "YScaleName"=w661, "Data Only"=w640) -> (w659:T1)
              n251 = Bundle By Name(cluster=w628, "GraphConfig"=w641) -> (w643:refnum<class "Interface.lvclass">)
              n252 = Replace Array Subset(array=w660, new element=w659, index=w618) -> (w617:T1[])
              n253 = Merge Errors(w642, w651, w627) -> (w652:errorcluster)
            }
            n254 = call "UpdateCurveSetup.vi"("ErrorIn(No Error)"=w609, "CurveSetupsIn"=w605, "Interface.lvclass"=w607) -> ("sortie d'erreur"=w608:errorcluster, "Interface.lvclass Out"=w606:refnum<class "Interface.lvclass">)  [unwired: 7 in]
          }
          frame "SaveParamsDef" {
            n255 = local read "2D Plot Act"() -> (w711:bool)
            n256 = local read "GraphIndex"() -> (w714:i32)
            n257 = Unbundle By Name(w718) -> ("XScalesNames"=w724:string[][], "YScalesNames"=w723:string[][])
            n258 = case shown="Vrai" w711 {
              tunnel: w712 -> [_ w768]
              tunnel: w691 -> [w765 w767]
              tunnel: [w765 w766] -> w709
              frame False {
              }
              frame True {
                n259 = Enqueue Element(queue=w768, element=SetupInterfStates."2D Graph" ("Énum"), error in (no error)=w767) -> (error out=w766:errorcluster)  [unwired: 1 in, 2 out]
              }
            }
            n260 = local read "YScaleName"() -> (w725:string)
            n261 = property on="X Scale" class="MDér (strict)"(error in=w691) -> (error out=w730:errorcluster, "Value"=w722:u32)  [unwired: 1 in, 1 out]
            n262 = local read "XScaleName"() -> (w726:string)
            n263 = property on="YScale" class="MDér (strict)"(error in=w730) -> (error out=w716:errorcluster, "Value"=w721:u32)  [unwired: 1 in, 1 out]
            n264 = Replace Array Subset(array=w723, new element=w725, index (row)=w714, index (col)=w721) -> (w719:string[][])
            n265 = Replace Array Subset(array=w724, new element=w726, index (row)=w714, index (col)=w722) -> (w720:string[][])
            n266 = Bundle By Name(cluster=T1 {"CurveName"="", "YParam"="", "XParam"="", "ZParam "="", "GroupName"="", "LinWdth"=1, "PntCol"=4294967295, "LinCol"=4294967295, "LablFor"=0, "XScale"=0, "YScale"=0, "Interpol"=2, "DisplayName"="", "FillType"=-1, "LineStyle"=0, "PntStyle"=12, "BarTyp"=0, "GraphIndex"=0, "Visible"=TRUE, "XScaleName"="", "YScaleName"="", "XYGraph_Ref"=refnum, "Data Only"=FALSE, "DataQ Ref"=refnum, "XParQ Ref"=refnum, "XParamInd"=0, "ScanInd"=0, "File Path"=path ""} ("CurveParam"), "XScale"=w722, "YScale"=w721, "GraphIndex"=w714) -> (w745:T1)
            n267 = Merge Errors(w709, w716) -> (w710:errorcluster)
            n268 = Bundle By Name(cluster=w718, "XScalesNames"=w720, "YScalesNames"=w719) -> (w717:refnum<class "Interface.lvclass">)
            n269 = property on="Graphe XY" class="GraphXY (strict)"(error in=w710, "Active Plot"=u32 0 ("Tracé actif")) -> (error out=w707:errorcluster, "Plot.Fill/Pt. Color"=w743:u32, "Plot.Plot Color"=w742:u32, "Plot.Line Width"=w752:u8, "Plot.Label Style"=w751:u8, "Plot.Plot Interpolation"=w750:u8, "Plot.Fill To"=w749:i16, "Plot.Line Style"=w748:u8, "Plot.Point Style"=w747:u8, "Plot.Bar Plot Style"=w746:u8)  [unwired: 1 in, 1 out]
            n270 = local read "AutoColor"() -> (w744:bool)
            n271 = call "SetGrphScale.vi"("error in (no error)"=w710, "GraphIndex"=w714, "Interface en entrée"=w717) -> ("error out"=w715:errorcluster, "Interface en sortie"=w698:refnum<class "Interface.lvclass">)  [unwired: 7 in]
            n272 = case shown="Vrai" w744 {
              tunnel: w745 -> [w775 w777]
              tunnel: w743 -> [w774 _]
              tunnel: w742 -> [w771 _]
              tunnel: [w773 w777] -> w736
              frame False {
                n273 = To Long Integer(number=w774) -> (32bit integer=w772:i32)
                n274 = To Long Integer(number=w771) -> (32bit integer=w770:i32)
                n275 = Bundle By Name(cluster=w775, "PntCol"=w772, "LinCol"=w770) -> (w773:T1)
              }
              frame True {
                w776 = -1 ("PntCol")
                n276 = Bundle By Name(cluster=w777, "PntCol"=w776, "LinCol"=w776) -> ()  [unwired: 1 out]
              }
            }
            n277 = local read "DisplayName"() -> (w708:string)
            n278 = Bundle By Name(cluster=w736, "LinWdth"=w752, "LablFor"=w751, "Interpol"=w750, "FillType"=w749, "LineStyle"=w748, "PntStyle"=w747, "BarTyp"=w746) -> (w738:T1)
            n279 = local read "VarParams"() -> (w734:string[][])
            n280 = local read "InstrPref"() -> (w704:string)
            n281 = property on="Curve List" class="LstDér (strict)"(error in=w707) -> (error out=w690:errorcluster, "Item Names"=w703:string[])  [unwired: 1 in, 1 out]
            n282 = property on="ScanParam" class="MDér (strict)"(error in=w707) -> (error out=w706:errorcluster, "Value"=w732:u16)  [unwired: 1 in, 1 out]
            n283 = local read "Visible"() -> (w741:bool)
            n284 = local read "XScaleName"() -> (w740:string)
            n285 = local read "YScaleName"() -> (w739:string)
            n286 = local read "Data Only"() -> (w727:bool)
            n287 = Index Array(array=w734, index (row)=0 ("indice (ligne)")) -> (element=w735:string[])  [unwired: 1 in]
            n288 = To Long Integer(number=w732) -> (32bit integer=w713:i32)
            n289 = Search 1D Array(1D array=w703, element=w704) -> (index of element=w693:i32)  [unwired: 1 in]
            n290 = Index Array(array=w735, index=w713) -> (element=w731:string)
            n291 = Greater Or Equal To 0?(x=w693) -> (x >= 0?=w700:bool)
            n292 = Bundle By Name(cluster=w738, "CurveName"=w704, "XParam"=w731, "XParamInd"=w713) -> (w737:T1)
            n293 = case shown="Faux" w700 {
              tunnel: w704 -> [w763 _]
              tunnel: w703 -> [w762 w764]
              tunnel: [w761 w764] -> w702
              frame False {
                n294 = Build Array (concatenate)(w762, w763) -> (w761:string[])
              }
              frame True {
              }
            }
            n295 = Bundle By Name(cluster=w737, "DisplayName"=w708, "Visible"=w741, "XScaleName"=w740, "YScaleName"=w739, "Data Only"=w727) -> (w701:T1)
            n296 = property on="Curve List" class="LstDér (strict)"(error in=w690, "Item Names"=w702) -> (error out=w705:errorcluster)  [unwired: 1 in, 1 out]
            n297 = case shown="Vrai" w700 {
              tunnel: w701 -> [w756 w759]
              tunnel: w692 -> [w755 w760]
              tunnel: [w754 w758] -> w694
              tunnel: w693 -> [_ w757]
              frame False {
                n298 = Build Array (concatenate)(w755, w756) -> (w754:T1[])
              }
              frame True {
                n299 = Replace Array Subset(array=w760, new element=w759, index=w757) -> (w758:T1[])
              }
            }
            n300 = Merge Errors(w705, w706, w715) -> (w696:errorcluster)
            n301 = local read "GraphConfig"() -> (w728:i32)
            n302 = call "UpdateCurveSetup.vi"("ErrorIn(No Error)"=w696, "CurveSetupsIn"=w694, "Interface.lvclass"=w698) -> ("sortie d'erreur"=w695:errorcluster, "Interface.lvclass Out"=w697:refnum<class "Interface.lvclass">)  [unwired: 7 in]
            n303 = Bundle By Name(cluster=w697, "GraphConfig"=w728) -> (w729:refnum<class "Interface.lvclass">)
          }
          frame "Stop" {
            n304 = control-ref of="ce VI"() -> (w781:refnum<vi>)
            n305 = property class="VI"(reference=w781, error in=w778) -> (error out=w779:errorcluster, "FP.State"=w780:T6)  [unwired: 1 out]
            n306 = case shown="\"Standard\", Par défaut" w780 {
              tunnel: [w786 w789] -> w782
              tunnel: w781 -> [_ w788]
              tunnel: w779 -> [w786 w787]
              frame "Closed" {
              }
              frame "Standard", Default {
                n307 = invoke class="VI" method="FA.Fermer"(reference=w788, error in=w787) -> (error out=w789:errorcluster)  [unwired: 1 in, 2 out]
              }
            }
          }
        }
      }
      n308 = while {
        shift-right: [w26] -> w12
        shift-left: w14 -> [w27]
        tunnel: w19 -> [w28]
        stop <- w24 stop-if-true
        n309 = event shown="[5] \"2D Plot\": Valeur changée" {
          selector: _ -> [_ _ _ _ _ _ _ _ _ _ _ _ _]
          dyn-events: _ -> [_ _ _ _ _ _ _ _ _ _ _ _ _]
          timeout: 200 -> [_ _ _ _ _ _ _ _ _ _ _ _ _]
          tunnel: w28 -> [_ w34 w39 w50 w62 _ _ _ w161 w188 w204 w208 w211]
          tunnel: w27 -> [w30 w36 w38 w49 w61 w81 w117 w159 w170 w190 w203 w207 w212]
          tunnel: [w30 w35 w37 w48 w60 w78 w122 w159 w162 w189 w192 w205 w209] -> w26
          tunnel: [_ TRUE _ _ _ _ _ _ _ _ _ _ _] -> w23
          event Timeout {
            n310 = event-data() -> ()  [unwired: 1 in, 2 out]
          }
          event "stop": Value Change; Panel Close {
            n311 = event-data() -> ()  [unwired: 1 in, 2 out]
            n312 = Enqueue Element(queue=w34, element=SetupInterfStates."Stop" ("Énum"), error in (no error)=w36) -> (error out=w35:errorcluster)  [unwired: 1 in, 2 out]
            n313 = local write "stop"(FALSE ("stop")) -> ()
          }
          event "SaveCurvePar": Value Change {
            n314 = event-data() -> ("NewVal"=w40:bool)  [unwired: 1 in, 4 out]
            n315 = case shown="Vrai" w40 {
              selector: w40 -> [_ w47]
              tunnel: w39 -> [_ w45]
              tunnel: w38 -> [w41 w44]
              tunnel: [w41 w43] -> w37
              frame False {
              }
              frame True {
                n316 = Not(x=w47) -> (.not. x?=w46:bool)
                n317 = local write "SaveCurvePar"(w46) -> ()
                n318 = Enqueue Element(queue=w45, element=SetupInterfStates."SaveParams" ("Énum"), error in (no error)=w44) -> (error out=w43:errorcluster)  [unwired: 1 in, 2 out]
              }
            }
          }
          event "SaveCurveParDef": Value Change {
            n319 = event-data() -> ("NewVal"=w51:bool)  [unwired: 1 in, 4 out]
            n320 = case shown="Vrai" w51 {
              selector: w51 -> [_ w58]
              tunnel: w50 -> [_ w56]
              tunnel: w49 -> [w52 w55]
              tunnel: [w52 w54] -> w48
              frame False {
              }
              frame True {
                n321 = Not(x=w58) -> (.not. x?=w57:bool)
                n322 = local write "SaveCurveParDef"(w57) -> ()
                n323 = Enqueue Element(queue=w56, element=SetupInterfStates."SaveParamsDef" ("Énum"), error in (no error)=w55) -> (error out=w54:errorcluster)  [unwired: 1 in, 2 out]
              }
            }
          }
          event "Apply All": Value Change {
            n324 = event-data() -> ("NewVal"=w63:bool)  [unwired: 1 in]
            n325 = case shown="Vrai" w63 {
              selector: w63 -> [w64 w72]
              tunnel: w62 -> [_ w71]
              tunnel: w61 -> [w65 w70]
              tunnel: [w65 w69] -> w60
              tunnel: [w64 w68] -> w59
              frame False {
              }
              frame True {
                n326 = Not(x=w72) -> (.not. x?=w68:bool)
                n327 = Two Button Dialog(message="This will apply current settings to all data items in curve list") -> (T button?=w66:bool)  [unwired: 2 in]
                n328 = case shown="Vrai" w66 {
                  tunnel: w71 -> [_ w77]
                  tunnel: w70 -> [w73 w76]
                  tunnel: [w73 w75] -> w69
                  frame False {
                  }
                  frame True {
                    n329 = Enqueue Element(queue=w77, element=SetupInterfStates."ApplyAll" ("Énum"), error in (no error)=w76) -> (error out=w75:errorcluster)  [unwired: 1 in, 2 out]
                  }
                }
              }
            }
            n330 = local write "Apply All"(w59) -> ()
          }
          event "2D Plot": Value Change {
            n331 = event-data() -> ("NewVal"=w82:bool)  [unwired: 1 in, 4 out]
            n332 = control-ref of="2D XScanPar"() -> (w80:refnum<vi>)
            n333 = control-ref of="2D YScanPar"() -> (w79:refnum<vi>)
            n334 = case shown="Vrai" w82 {
              tunnel: w81 -> [w94 w110]
              tunnel: w80 -> [w93 w109]
              tunnel: w79 -> [_ w108]
              tunnel: [w87 w100] -> w78
              frame True {
                n335 = Build Array(w93) -> (w96:refnum<vi>[])
                n336 = call <userlib>:"SetCtrlPropGen.vi"("Error in"=w94, "Énum"=T3."Enable", "Controls"=w96) -> ("Error out"=w83:errorcluster)  [unwired: 3 in, 1 out]
                n337 = local read "VarParams"() -> (w92:string[][])
                n338 = call <userlib>:"ArrayTo1DString.vi"("ErrorIn(No Error)"=w83, "DelArrEnd(F)"=TRUE ("DelArrEnd"), "tableau"=w92) -> ("sortie d'erreur"=w84:errorcluster, "Array Out"=w86:string[])  [unwired: 6 in, 1 out]
                n339 = for {
                  tunnel: w86 -> [w99] mode=indexing
                  tunnel: [w98] -> w85 mode=indexing
                  n340 = Match Pattern(string=w99, regular expression="_" ("expression régulière")) -> (before substring=w98:string)  [unwired: 1 in, 3 out]
                }
                n341 = Build Array (concatenate)("Selectionner un Paramètre.." ("PanelIndex"), w85) -> (w89:string[])
                n342 = property on="2D XScanPar" class="MDér (strict)"(error in=w84, "Strings []"=w89) -> (error out=w90:errorcluster)  [unwired: 1 in, 1 out]
                n343 = Merge Errors(w83, w90) -> (w87:errorcluster)
              }
              frame False {
                n344 = Build Array(w109, w108) -> (w102:refnum<vi>[])
                n345 = call <userlib>:"SetCtrlPropGen.vi"("Error in"=w110, "Énum"=T3."DisAndGrayed", "Controls"=w102) -> ("Error out"=w107:errorcluster, "Controls Out"=w106:refnum<vi>[])  [unwired: 3 in]
                n346 = call <userlib>:"SetCtrlPropGen.vi"("Error in"=w107, "Énum"=T4."EnumElementsArr", "Controls"=w106) -> ("Error out"=w104:errorcluster, "Controls Out"=w103:refnum<vi>[])  [unwired: 3 in]
                n347 = call <userlib>:"SetCtrlPropGen.vi"("Error in"=w104, "Énum"=T4."ReinitToDefVal", "Controls"=w103) -> ("Error out"=w100:errorcluster)  [unwired: 3 in, 1 out]
              }
            }
          }
          event "2D XScanPar": Value Change {
            n348 = event-data() -> ()  [unwired: 1 in, 1 out]
            n349 = control-ref of="2D YScanPar"() -> (w127:refnum<vi>)
            n350 = property on="2D XScanPar" class="MDér (strict)"(error in=w117) -> (error out=w130:errorcluster, "RingText.Text"=w133:string)  [unwired: 1 in, 1 out]
            n351 = local read "VarParams"() -> (w112:string[][])
            n352 = for {
              tunnel: w112 -> [w150] mode=indexing
              tunnel: w133 -> [w154]
              tunnel: [w152] -> w119
              i -> [w152]
              stop <- w151 stop-if-true
              n353 = for {
                tunnel: w150 -> [w157] mode=indexing
                tunnel: [w156] -> w149 mode=indexing
                n354 = Match Pattern(string=w157, regular expression="_" ("expression régulière")) -> (before substring=w156:string)  [unwired: 1 in, 3 out]
              }
              n355 = Search 1D Array(1D array=w149, element=w154) -> (index of element=w153:i32)  [unwired: 1 in]
              n356 = Greater Or Equal To 0?(x=w153) -> (x >= 0?=w151:bool)
            }
            n357 = Build Array(w127) -> (w128:refnum<vi>[])
            n358 = property on="2D YScanPar" class="MDér (strict)"(error in=w117) -> (error out=w116:errorcluster, "Value"=w118:u16)  [unwired: 1 in, 1 out]
            n359 = call <userlib>:"SetCtrlPropGen.vi"("Error in"=w130, "Énum"=T3."Enable", "Controls"=w128) -> ("Error out"=w129:errorcluster)  [unwired: 3 in, 1 out]
            n360 = Equal To 0?(x=w119) -> (x = 0?=→"Fill Line First":bool)
            n361 = Delete From Array(array=w112, index (row)=w119) -> (array with subset deleted=w132:string[][])  [unwired: 2 in, 1 out]
            n362 = Equal To 0?(x=w118) -> (x = 0?=w114:bool)
            n363 = call <userlib>:"ArrayTo1DString.vi"("ErrorIn(No Error)"=w129, "DelArrEnd(F)"=TRUE ("DelArrEnd"), "tableau"=w132) -> ("sortie d'erreur"=w126:errorcluster, "Array Out"=w115:string[])  [unwired: 6 in, 1 out]
            n364 = case shown="Faux" w114 {
              tunnel: w112 -> [w143 _]
              tunnel: w118 -> [w141 w145]
              tunnel: w116 -> [w140 _]
              tunnel: w115 -> [w138 _]
              tunnel: [w134 w145] -> w113
              frame False {
                n365 = call <userlib>:"ArrayTo1DString.vi"("ErrorIn(No Error)"=w140, "DelArrEnd(F)"=TRUE ("DelArrEnd"), "tableau"=w143) -> ("Array Out"=w142:string[])  [unwired: 6 in, 2 out]
                n366 = To Long Integer(number=w141) -> (32bit integer=w139:i32)
                n367 = Index Array(array=w142, index=w139) -> (element=w137:string)
                n368 = Search 1D Array(1D array=w138, element=w137) -> (index of element=w136:i32)  [unwired: 1 in]
                n369 = To Unsigned Word Integer(number=w136) -> (unsigned 16bit integer=w135:u16)
                n370 = Increment(x=w135) -> (x+1=w134:u16)
              }
              frame True {
              }
            }
            n371 = for {
              tunnel: w115 -> [w148] mode=indexing
              tunnel: [w147] -> w121 mode=indexing
              n372 = Match Pattern(string=w148, regular expression="_" ("expression régulière")) -> (before substring=w147:string)  [unwired: 1 in, 3 out]
            }
            n373 = Build Array (concatenate)("Selectionner un Paramètre.." ("PanelIndex"), w121) -> (w124:string[])
            n374 = property on="2D YScanPar" class="MDér (strict)"(error in=w126, "Strings []"=w124, "Value"=w113) -> (error out=w122:errorcluster)  [unwired: 1 in, 1 out]
          }
          event "2D YScanPar": Value Change {
            n375 = event-data() -> ("NewVal"=w160:u16)  [unwired: 1 in, 4 out]
            n376 = Greater Than 0?(x=w160) -> (x > 0?=w158:bool)
            n377 = local write "2D Plot Act"(w158) -> ()
          }
          event "Graph Window": Value Change {
            n378 = event-data() -> ("NewVal"=w165:i32)  [unwired: 1 in, 4 out]
            n379 = property on="Graph Window" class="MDér (strict)"() -> ("Strings []"=w172:string[])  [unwired: 2 in, 2 out]
            n380 = Index Array(array=w172, index=w165) -> (element=w167:string)
            n381 = Scan From String(format string="Graph %d" ("chaîne de format"), input string=w167, error in=w170) -> (error out=w169:errorcluster, output 1=w168:i32)  [unwired: 2 in, 2 out]
            n382 = case shown="Erreur" w169 {
              selector: w169 -> [w173 w184]
              tunnel: w168 -> [w174 _]
              tunnel: w167 -> [_ w181]
              tunnel: [w174 w185] -> w166
              tunnel: [w173 w183] -> w163
              frame No Error {
              }
              frame Error {
                n383 = Match Pattern(string=w181, regular expression="Scan" ("expression régulière")) -> (offset past match=w179:i32)  [unwired: 1 in, 3 out]
                n384 = Greater Than 0?(x=w179) -> (x > 0?=w178:bool)
                n385 = Equal?(x=w181, y="No Graph") -> (x = y?=w182:bool)
                n386 = Select(t=-3 ("GraphIndex"), s=w178, f=-1 ("GraphIndex")) -> (s? t:f=w175:i32)
                n387 = call <vilib>:"Clear Errors.vi"("error in (no error)"=w184) -> ("error out"=w183:errorcluster)  [unwired: 5 in, 1 out]
                n388 = Select(t=-2 ("GraphIndex"), s=w182, f=w175) -> (s? t:f=w185:i32)
                n389 = local write "Data Only"(w182) -> ()
              }
            }
            n390 = local write "GraphIndex"(w166) -> ()
            n391 = Enqueue Element(queue=w161, element=SetupInterfStates."GetScaleName" ("Énum"), error in (no error)=w163) -> (error out=w162:errorcluster)  [unwired: 1 in, 2 out]
          }
          event "ScanParam": Value Change {
            n392 = event-data() -> ()  [unwired: 1 in, 5 out]
            n393 = Enqueue Element(queue=w188, element=SetupInterfStates."GetScaleName" ("Énum"), error in (no error)=w190) -> (error out=w189:errorcluster)  [unwired: 1 in, 2 out]
          }
          event "Curve List": Value Change {
            n394 = event-data() -> ()  [unwired: 1 in, 5 out]
            n395 = Enqueue Element(queue=w204, element=SetupInterfStates."ReadMeasPar" ("élément"), error in (no error)=w203) -> (queue out=w200:refnum<queue>, error out=w201:errorcluster)  [unwired: 1 in, 1 out]
            n396 = Enqueue Element(queue=w200, element=SetupInterfStates."ReadCurvePar" ("élément"), error in (no error)=w201) -> (queue out=w197:refnum<queue>, error out=w198:errorcluster)  [unwired: 1 in, 1 out]
            n397 = Enqueue Element(queue=w197, element=SetupInterfStates."ReadGraphPar" ("élément"), error in (no error)=w198) -> (queue out=w193:refnum<queue>, error out=w194:errorcluster)  [unwired: 1 in, 1 out]
            n398 = Enqueue Element(queue=w193, element=SetupInterfStates."GetScaleName" ("Énum"), error in (no error)=w194) -> (error out=w192:errorcluster)  [unwired: 1 in, 2 out]
          }
          event "XScaleName", "YScaleName": Value Change {
            n399 = event-data() -> ()  [unwired: 1 in, 5 out]
            n400 = Enqueue Element(queue=w208, element=SetupInterfStates."ChgScaleName" ("Énum"), error in (no error)=w207) -> (error out=w205:errorcluster)  [unwired: 1 in, 2 out]
          }
          event "X Scale", "YScale": Value Change {
            n401 = event-data() -> ()  [unwired: 1 in, 5 out]
            n402 = Enqueue Element(queue=w211, element=SetupInterfStates."GetScaleName" ("Énum"), error in (no error)=w212) -> (error out=w209:errorcluster)  [unwired: 1 in, 2 out]
          }
        }
        n403 = Or(x=w23, y="stop") -> (x .or. y?=w24:bool)
      }
      n404 = Merge Errors(w11, w12) -> (w10:errorcluster)
    }
    frame Error {
    }
  }
  "error out" <- w5
  "Interface en sortie" <- w3
  "CurveParamsOut" <- w1
